vi "Main.vi"() -> ()   [LabVIEW 2019]
uses:
  03 DQMH Modules/SME_Data_Acquisition/SME_Data_Acquisition.lvlib
  03 DQMH Modules/SME_Report/SME_Report.lvlib
panel:
  out "MainTitle":string="SME Client Application"
  in  "Close":bool
  in  "Analysis":bool
  in  "DAQ":bool
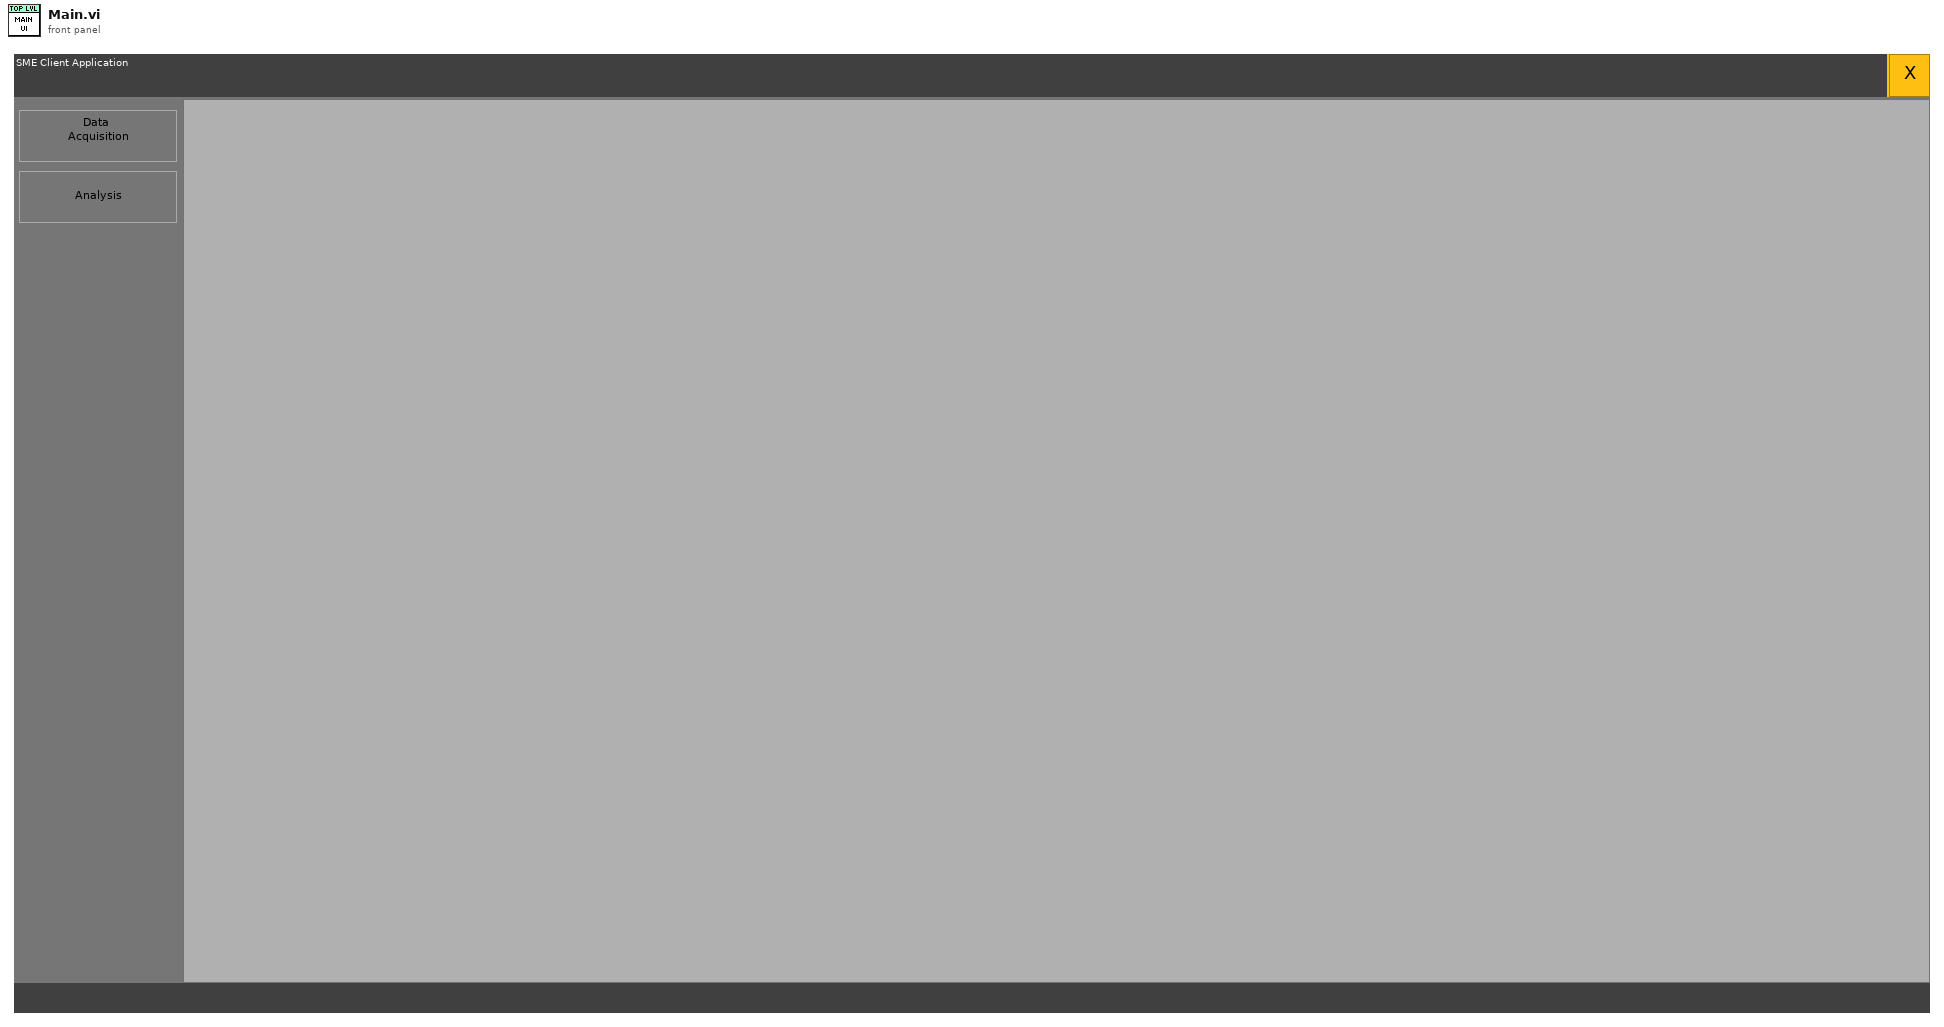
[diagram p1: front panel]
types:
  T1 = enum32{"Invalid", "Standard", "Closed", "Hidden", "Minimized", "Maximized"}
  T2 = enum32{"invalid app kind", "Development System", "Run Time System", "Student Edition", "Embedded LabVIEW", "Evaluation", "Custom"}
  T3 = cluster{"Core":cluster{"Current VI Reference":refnum<vi>, "Close Panel on Exit?":bool}, "MainTitle":refnum<vi>, "SubPanel":refnum<vi>}
  T4 = cluster{"Current VI Reference":refnum<vi>, "Close Panel on Exit?":bool}
  T5 = typedef "LVRectTypeDef.ctl" = cluster{"Left":i16, "Top":i16, "Right":i16, "Bottom":i16}
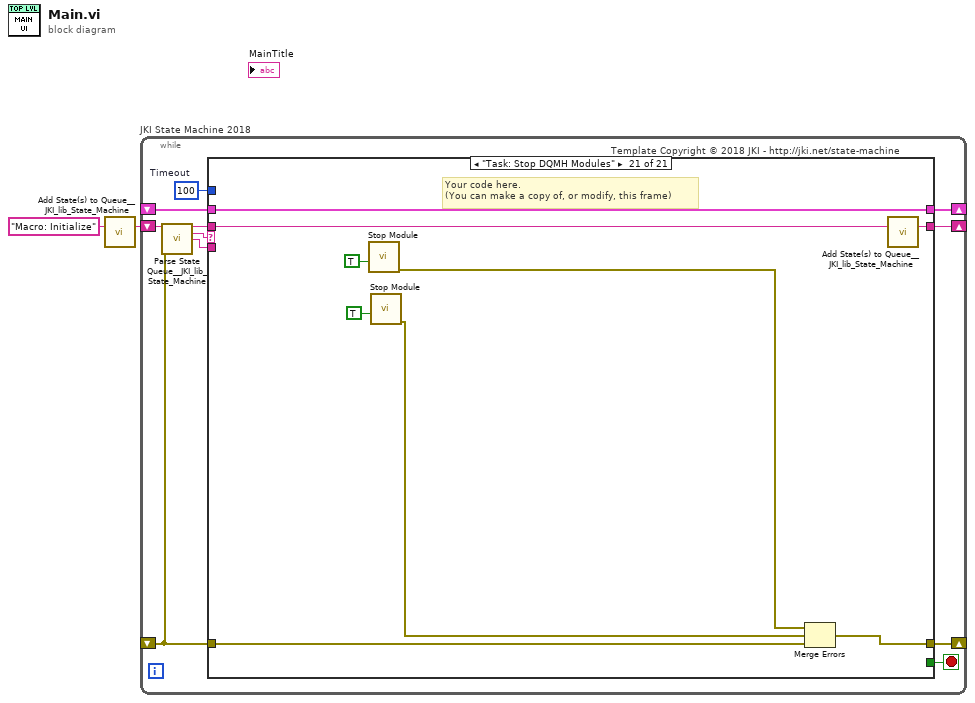
[diagram p0: block diagram]
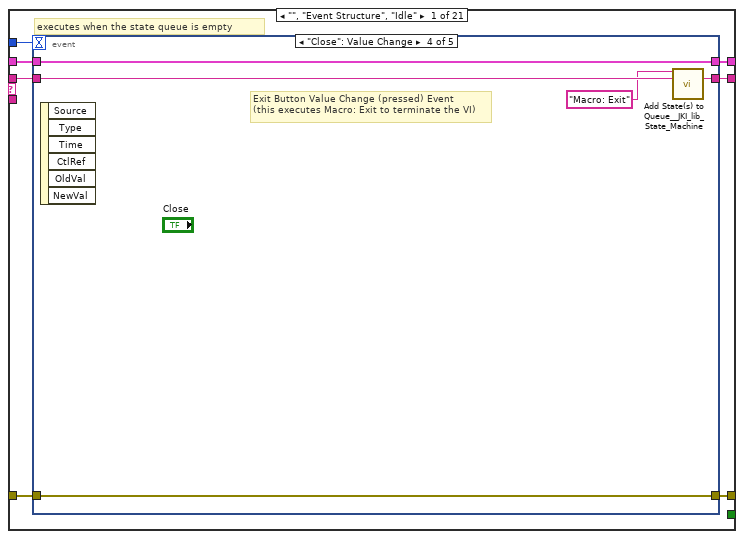
[diagram p2: hidden frame]
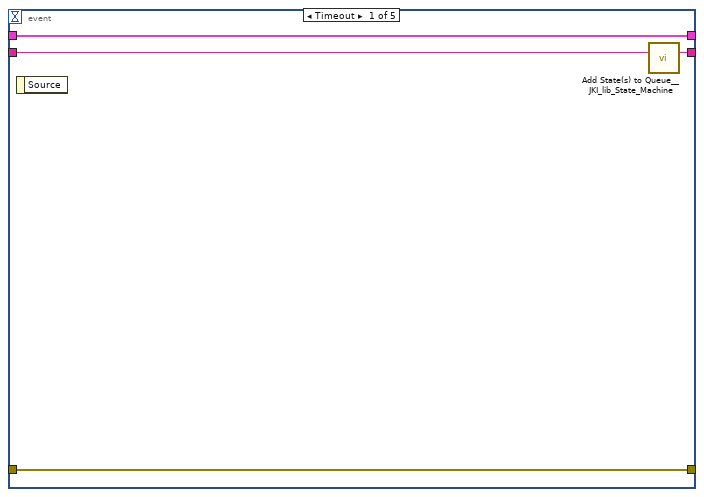
[diagram p3: hidden frame]
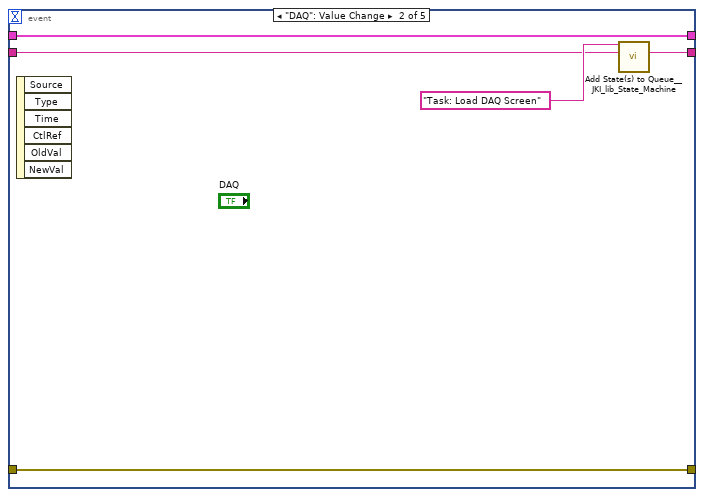
[diagram p4: hidden frame]
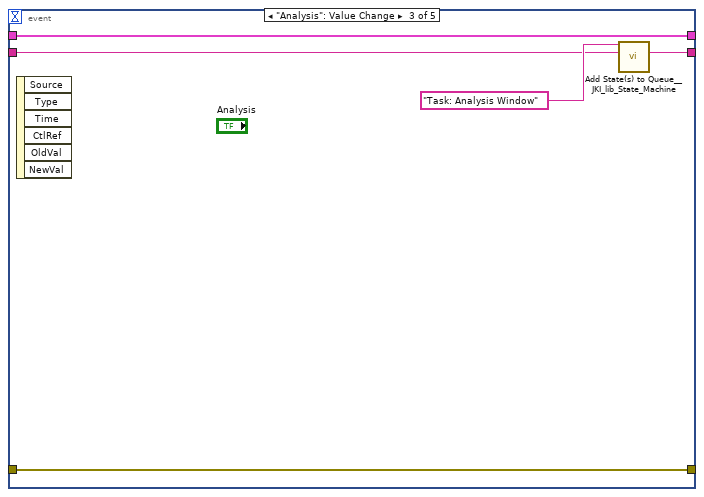
[diagram p5: hidden frame]
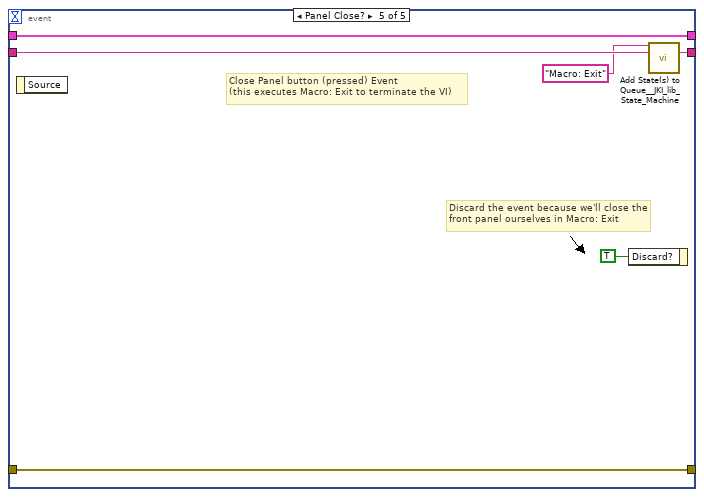
[diagram p6: hidden frame]
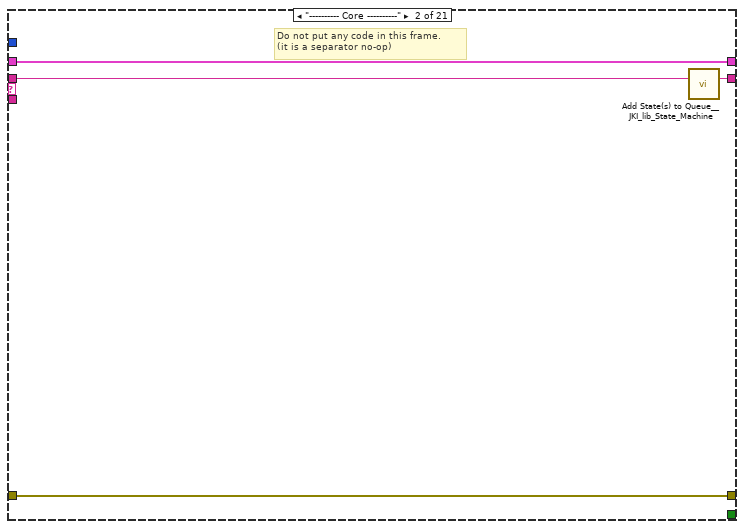
[diagram p7: hidden frame]
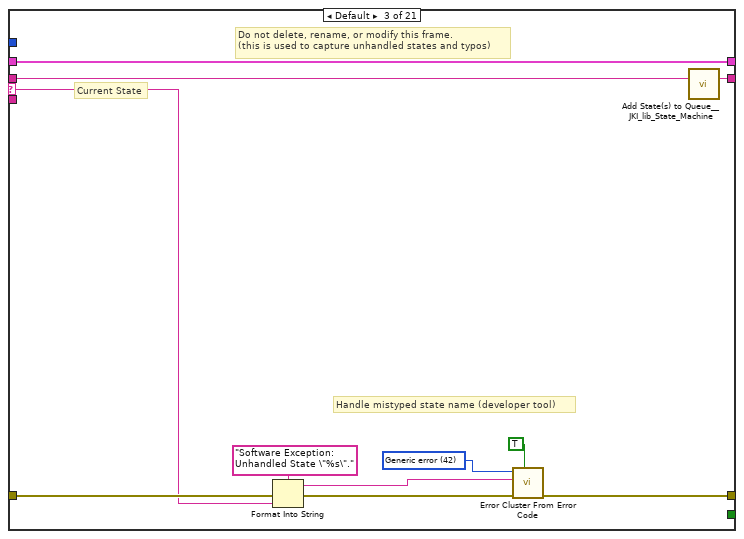
[diagram p8: hidden frame]
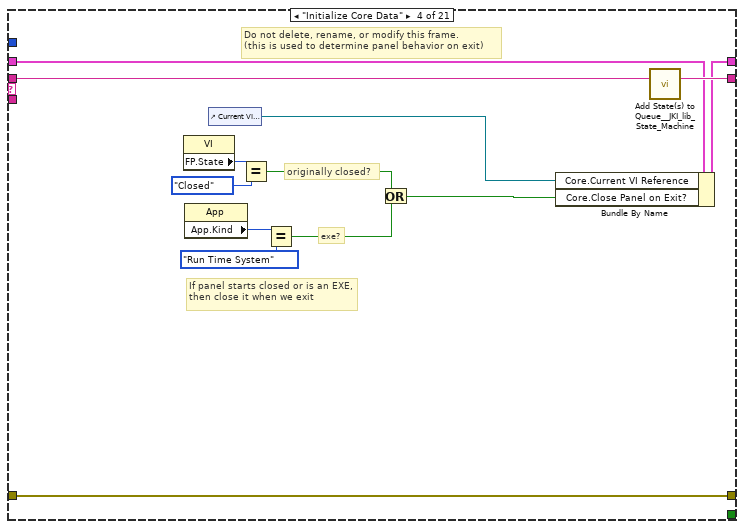
[diagram p9: hidden frame]
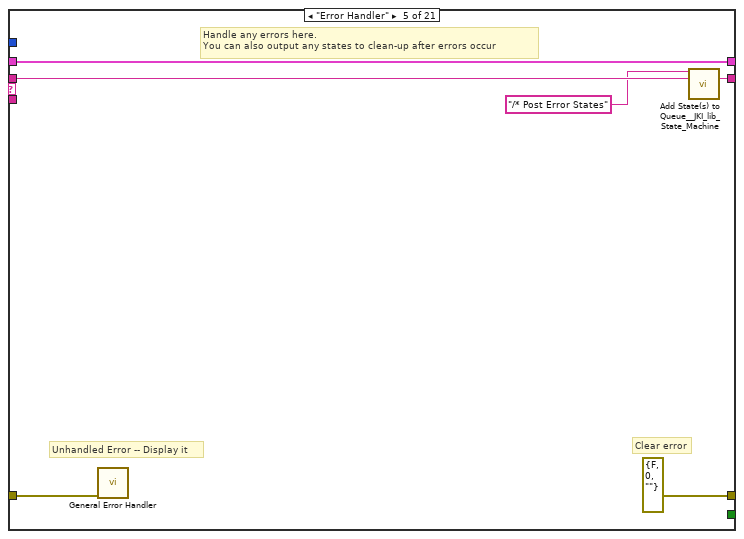
[diagram p10: hidden frame]
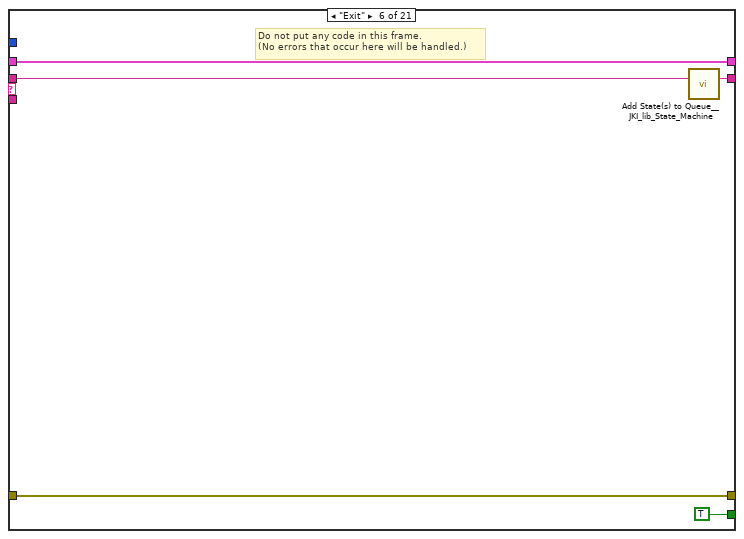
[diagram p11: hidden frame]
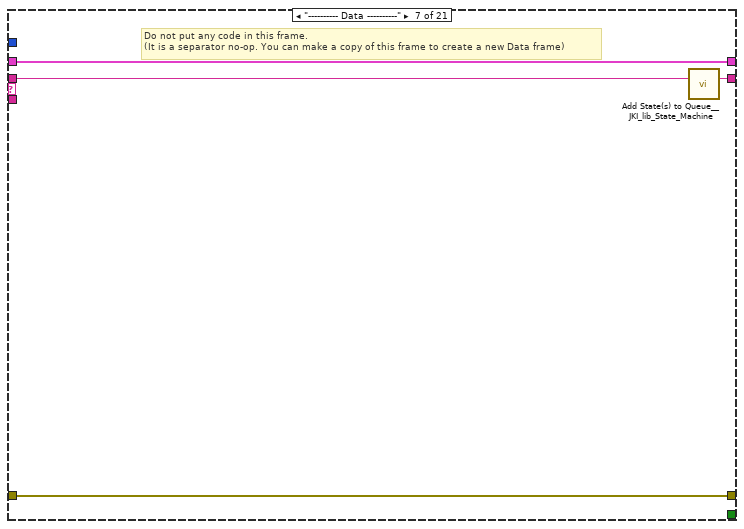
[diagram p12: hidden frame]
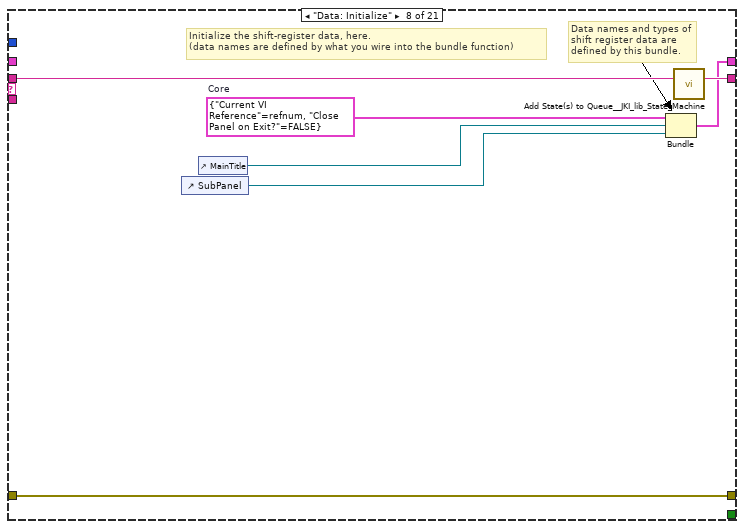
[diagram p13: hidden frame]
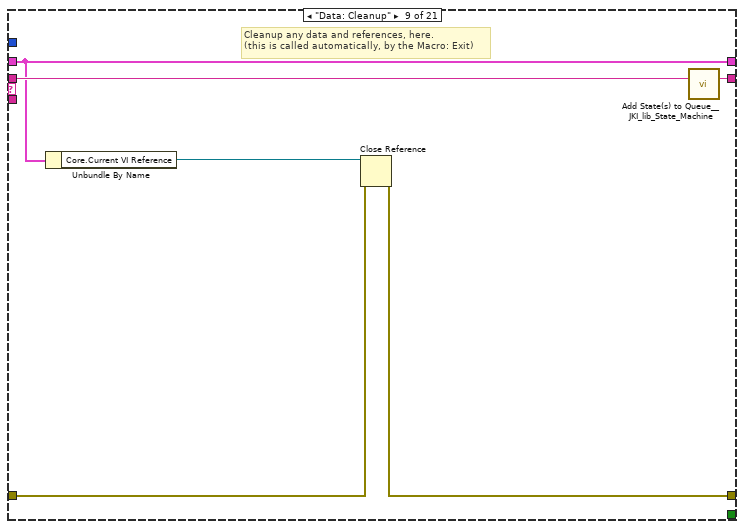
[diagram p14: hidden frame]
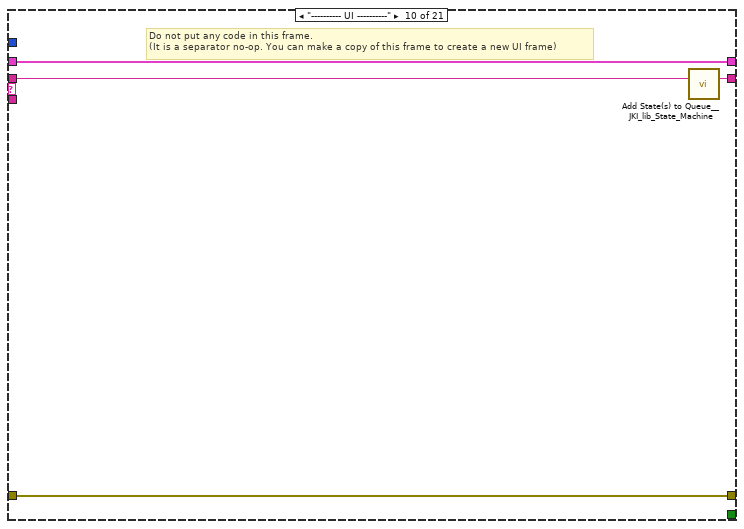
[diagram p15: hidden frame]
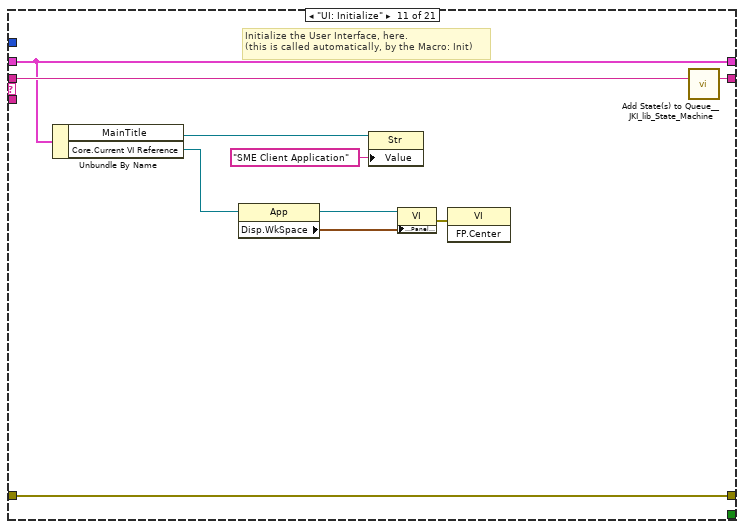
[diagram p16: hidden frame]
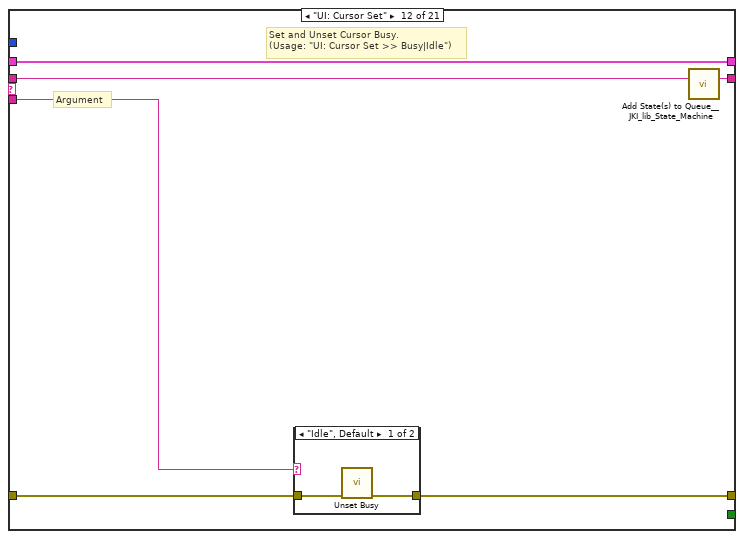
[diagram p17: hidden frame]
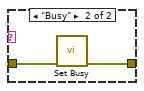
[diagram p18: hidden frame]
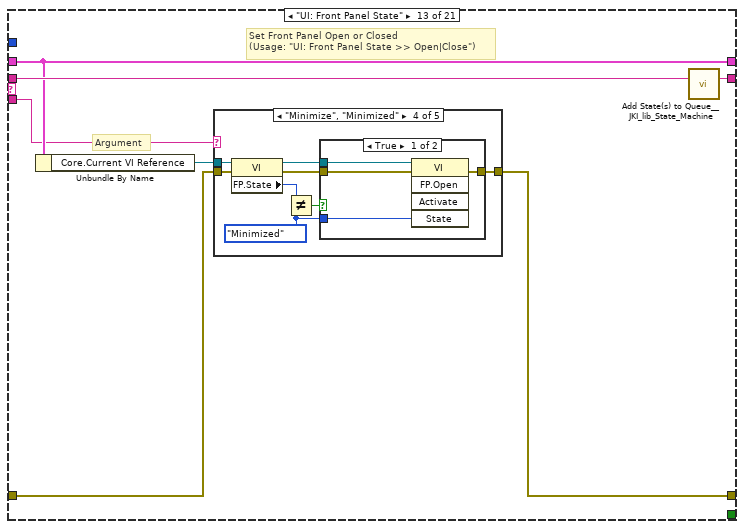
[diagram p19: hidden frame]
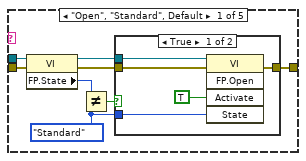
[diagram p20: hidden frame]
diagram:
  n1 = call <vilib>:"Add State(s) to Queue__JKI_lib_State_Machine.vi"("State(s) in (\"\")"="Macro: Initialize") -> ("States Out"=w2:string)  [unwired: 14 in]
  n2 = while "JKI State Machine 2018" {
    shift-right: [w6] -> _
    shift-left: _ -> [w5]
    shift-right: [w9] -> _
    shift-left: _ -> [w3]
    shift-right: [w8] -> _
    shift-left: w2 -> [w10]
    stop <- w7 stop-if-true
    w4 = 100  # Timeout
    # "Template Copyright © 2018 JKI - http://jki.net/state-machine"
    n3 = call <vilib>:"Parse State Queue__JKI_lib_State_Machine.vi"("State Queue"=w10, "Error In (no error)"=w3) -> ("Remaining States"=w12:string, "Current State"=w13:string, "Arguments"=w11:string)  [unwired: 11 in]
    n4 = case shown="\"Task: Stop DQMH Modules\"" w13 {
      selector: w13 -> [_ _ w50 _ _ _ _ _ _ _ _ _ _ _ _ _ _ _ _ _ _]
      tunnel: w12 -> [w20 w49 w54 w73 w79 w84 w88 w95 w101 w105 w114 w120 w131 w200 w205 w215 w219 w230 w240 w250 w259]
      tunnel: w11 -> [_ _ _ _ _ _ _ _ _ _ _ w115 w125 _ _ _ _ _ _ _ _]
      tunnel: w5 -> [w18 w46 w52 w66 w76 w82 w85 _ w96 w102 w111 w118 w127 w197 w203 w212 w216 w227 w231 w248 w256]
      tunnel: [w17 w47 w56 w70 errorcluster {"status"=FALSE, "code"=0, "source"=""} ("error out") w81 w86 w92 w97 w103 w112 w116 w128 w198 w201 w213 w217 w224 w238 w247 w255] -> w9
      tunnel: w3 -> [w16 w47 w55 w70 w75 w81 w86 w92 w98 w103 w112 w117 w129 w198 w201 w213 w217 w228 w238 w246 w257]
      tunnel: [w19 w48 w53 w72 w78 w83 w87 w94 w100 w104 w113 w119 w130 w199 w204 w214 w218 w229 w239 w249 w258] -> w8
      tunnel: [_ _ _ _ _ TRUE _ _ _ _ _ _ _ _ _ _ _ _ _ _ _] -> w7
      tunnel: [w15 w46 w52 w71 w76 w82 w85 w93 w96 w102 w111 w118 w127 w197 w203 w212 w216 w227 w231 w248 w256] -> w6
      tunnel: w4 -> [w14 _ _ _ _ _ _ _ _ _ _ _ _ _ _ _ _ _ _ _ _]
      frame "", "Event Structure", "Idle" {
        # "executes when the state queue is empty"
        n5 = event shown="[3] \"Close\": Value Change" {
          selector: _ -> [_ _ _ _ _]
          dyn-events: _ -> [_ _ _ _ _]
          timeout: w14 -> [_ _ _ _ _]
          tunnel: w20 -> [w24 w26 w31 w39 w45]
          tunnel: [w23 w27 w32 w38 w44] -> w19
          tunnel: w18 -> [w21 w29 w34 w36 w42]
          tunnel: [w22 w25 w30 w37 w43] -> w17
          tunnel: w16 -> [w22 w25 w30 w37 w43]
          tunnel: [w21 w29 w34 w36 w42] -> w15
          event Timeout {
            n6 = event-data() -> ()  [unwired: 1 in, 1 out]
            n7 = call <vilib>:"Add State(s) to Queue__JKI_lib_State_Machine.vi"("State(s) in (\"\")"=w24) -> ("States Out"=w23:string)  [unwired: 14 in]
          }
          event "DAQ": Value Change {
            n8 = event-data() -> ()  [unwired: 1 in, 6 out]
            n9 = call <vilib>:"Add State(s) to Queue__JKI_lib_State_Machine.vi"("State(s) in Front (\"\")"="Task: Load DAQ Screen", "State(s) in (\"\")"=w26) -> ("States Out"=w27:string)  [unwired: 13 in]
          }
          event "Analysis": Value Change {
            n10 = event-data() -> ()  [unwired: 1 in, 6 out]
            n11 = call <vilib>:"Add State(s) to Queue__JKI_lib_State_Machine.vi"("State(s) in Front (\"\")"="Task: Analysis Window", "State(s) in (\"\")"=w31) -> ("States Out"=w32:string)  [unwired: 13 in]
          }
          event "Close": Value Change {
            # "Exit Button Value Change (pressed) Event\n(this executes Macro: Exit to terminate the VI)"
            n12 = event-data() -> ()  [unwired: 1 in, 6 out]
            n13 = call <vilib>:"Add State(s) to Queue__JKI_lib_State_Machine.vi"("State(s) in Front (\"\")"="Macro: Exit", "State(s) in (\"\")"=w39) -> ("States Out"=w38:string)  [unwired: 13 in]
          }
          event Panel Close? {
            # "Discard the event because we'll close the front panel ourselves in Macro: Exit"
            # "Close Panel button (pressed) Event\n(this executes Macro: Exit to terminate the VI)"
            n14 = event-data() -> ()  [unwired: 1 in, 1 out]
            n15 = event-data("Discard?"=TRUE) -> ()  [unwired: 1 in, 1 out]
            n16 = call <vilib>:"Add State(s) to Queue__JKI_lib_State_Machine.vi"("State(s) in Front (\"\")"="Macro: Exit", "State(s) in (\"\")"=w45) -> ("States Out"=w44:string)  [unwired: 13 in]
          }
        }
      }
      frame "---------- Core ----------" {
        # "Do not put any code in this frame.\n(it is a separator no-op)"
        n17 = call <vilib>:"Add State(s) to Queue__JKI_lib_State_Machine.vi"("State(s) in (\"\")"=w49) -> ("States Out"=w48:string)  [unwired: 14 in]
      }
      frame Default {
        w59 = 42 items=["No error", "Argument error", "Memory is full", "Out of zone", "End of file", "File already open", "Generic file I/O error", "File not found", "File permission error", "Disk is full", "Duplicate path", "Too many files open", "System feature not enabled", "Resource file not found", "Cannot add resource", "Resource not found", "Image not found", "Image memory error", "Pen does not exist", "Config type invalid", "Config token not found", "Config parse error", "Config memory error", "Bad external code format", "Bad external code offset", "External code not present", "Null window", "Destroy window error", "Null menu", "Print aborted", "Bad print record", "Print driver error", "Windows error during printing", "Memory error during printing", "Print dialog error", "Generic print error", "Invalid device refnum", "Device not found", "Device parameter error", "Device unit error", "Cannot open device", "Device call aborted", "Generic error", "Cancelled by user", "Object ID too low", "Object ID too high", "Object not in heap", "Unknown heap", "Unknown object (invalid DefProc)", "Unknown object (DefProc not in table)", "Message out of range", "Invalid (null) method", "Unknown message", "Manager call not supported", "Bad address", "Network operation in progress", "Network operation timed out", "Connection is busy", "Network attribute not supported", "Network error", "Address in use", "System out of memory", "Connection aborted", "Connection refused", "Not connected", "Already connected", "Connection closed", "Initialization error (interapplication manager)", "Bad occurrence", "Wait on unbound occurrence handler", "Occurrence queue overflow", "Datalog type conflict", "Unused", "Unrecognized type (interapplication manager)", "Memory corrupt", "Failed to make temporary DLL", "Old CIN version", "Drag socket not found", "Failed to load drop-object", "Failed to register OLE object", "Failed to release OLE object", "Format specifier type mismatch", "Unknown format specifier", "Too few format specifiers", "Too many format specifiers", "Scan failed", "Newer CIN version", "Error converting to variant", "Runtime menu error", "Password tampered", "Variant attribute not found", "Incompatible variant data type", "Event data is not available", "Event Store is not present", "Occurrence is not found", "Event Queue is not created", "Event info is not available", "Refnum passed is NULL", "Error retrieving Class GUID", "Error retrieving CoClass GUID", "Error retrieving TypeLib GUID.", "Bad built application magic bytes.", "Specific driver is different from the specific driver associated with the Logical Name.", "There is no session opened to the class driver.", "Max Error", "MAX - Error with config objects", "MAX - Error loading configuration", "MAX - Group not supported"]
        # "Current State"
        # "Do not delete, rename, or modify this frame.\n(this is used to capture unhandled states and typos)"
        # "Handle mistyped state name (developer tool)"
        n18 = Format Into String(format string="Software Exception: Unhandled State \"%s\"." ("message"), error in=w55, w50) -> (resulting string=w58:string, error out=w57:errorcluster)  [unwired: 1 in]
        n19 = call <vilib>:"Error Cluster From Error Code.vi"("show call chain? (False)"=TRUE, "error in (no error)"=w57, "error message (\"\")"=w58, "error code (0)"=w59) -> ("error out"=w56:errorcluster)  [unwired: 5 in]
        n20 = call <vilib>:"Add State(s) to Queue__JKI_lib_State_Machine.vi"("State(s) in (\"\")"=w54) -> ("States Out"=w53:string)  [unwired: 14 in]
      }
      frame "Initialize Core Data" {
        # "Do not delete, rename, or modify this frame.\n(this is used to determine panel behavior on exit)"
        # "originally closed?"
        # "exe?"
        # "If panel starts closed or is an EXE, then close it when we exit"
        n21 = property class="VI"() -> ("FP.State"=w63:T1)  [unwired: 2 in, 2 out]
        n22 = property class="App"() -> ("App.Kind"=w69:T2)  [unwired: 2 in, 2 out]
        n23 = control-ref of="Current VI Reference"() -> (w64:refnum<vi>)
        n24 = Equal?(x=w63, y=T1."Closed" ("Front Panel Window:State")) -> (x = y?=w61:bool)
        n25 = Equal?(x=w69, y=T2."Run Time System" ("Application:Kind")) -> (x = y?=w67:bool)
        n26 = Or(x=w61, y=w67) -> (x .or. y?=w65:bool)
        n27 = Bundle By Name(cluster=w66, "Core.Current VI Reference"=w64, "Core.Close Panel on Exit?"=w65) -> (w71:T3)
        n28 = call <vilib>:"Add State(s) to Queue__JKI_lib_State_Machine.vi"("State(s) in (\"\")"=w73) -> ("States Out"=w72:string)  [unwired: 14 in]
      }
      frame "Error Handler" {
        # "Unhandled Error -- Display it"
        # "Handle any errors here.\nYou can also output any states to clean-up after errors occur"
        # "Clear error"
        n29 = call <vilib>:"General Error Handler.vi"("error in (no error)"=w75) -> ()  [unwired: 10 in, 5 out]
        n30 = call <vilib>:"Add State(s) to Queue__JKI_lib_State_Machine.vi"("State(s) in Front (\"\")"="/* Post Error States", "State(s) in (\"\")"=w79) -> ("States Out"=w78:string)  [unwired: 13 in]
      }
      frame "Exit" {
        # "Do not put any code in this frame.\n(No errors that occur here will be handled.)"
        n31 = call <vilib>:"Add State(s) to Queue__JKI_lib_State_Machine.vi"("State(s) in (\"\")"=w84) -> ("States Out"=w83:string)  [unwired: 14 in]
      }
      frame "---------- Data ----------" {
        # "Do not put any code in this frame.\n(It is a separator no-op. You can make a copy of this frame to create a new Data frame)"
        n32 = call <vilib>:"Add State(s) to Queue__JKI_lib_State_Machine.vi"("State(s) in (\"\")"=w88) -> ("States Out"=w87:string)  [unwired: 14 in]
      }
      frame "Data: Initialize" {
        w91 = T4 {"Current VI Reference"=refnum, "Close Panel on Exit?"=FALSE}  # Core
        # "Data names and types of shift register data are defined by this bundle."
        # "Initialize the shift-register data, here.\n(data names are defined by what you wire into the bundle function)"
        n33 = control-ref of="SubPanel"() -> (w90:refnum<vi>)
        n34 = control-ref of="MainTitle"() -> (w89:refnum<vi>)
        n35 = Bundle("Core"=w91, "MainTitle"=w89, "SubPanel"=w90) -> (w93:T3)  [unwired: 1 in]
        n36 = call <vilib>:"Add State(s) to Queue__JKI_lib_State_Machine.vi"("State(s) in (\"\")"=w95) -> ("States Out"=w94:string)  [unwired: 14 in]
      }
      frame "Data: Cleanup" {
        # "Cleanup any data and references, here.\n(this is called automatically, by the Macro: Exit)"
        n37 = Unbundle By Name(w96) -> ("Core.Current VI Reference"=w99:refnum<vi>)
        n38 = Close Reference(reference=w99, error in (no error)=w98) -> (error out=w97:errorcluster)
        n39 = call <vilib>:"Add State(s) to Queue__JKI_lib_State_Machine.vi"("State(s) in (\"\")"=w101) -> ("States Out"=w100:string)  [unwired: 14 in]
      }
      frame "---------- UI ----------" {
        # "Do not put any code in this frame.\n(It is a separator no-op. You can make a copy of this frame to create a new UI frame)"
        n40 = call <vilib>:"Add State(s) to Queue__JKI_lib_State_Machine.vi"("State(s) in (\"\")"=w105) -> ("States Out"=w104:string)  [unwired: 14 in]
      }
      frame "UI: Initialize" {
        # "Initialize the User Interface, here.\n(this is called automatically, by the Macro: Init)"
        n41 = Unbundle By Name(w111) -> ("MainTitle"=w110:refnum<vi>, "Core.Current VI Reference"=w106:refnum<vi>)
        n42 = property on="Property Node" class="App"() -> ("Disp.WkSpace"=w107:T5)  [unwired: 2 in, 2 out]
        n43 = property class="Str"(reference=w110, "Value"="SME Client Application") -> ()  [unwired: 1 in, 2 out]
        n44 = property on="Property Node" class="VI"(reference=w106, "Front Panel.PanelBounds"=w107) -> (error out=w108:errorcluster)  [unwired: 1 in, 1 out]
        n45 = invoke class="VI" method="FP.Center"(error in=w108) -> ()  [unwired: 2 in, 3 out]
        n46 = call <vilib>:"Add State(s) to Queue__JKI_lib_State_Machine.vi"("State(s) in (\"\")"=w114) -> ("States Out"=w113:string)  [unwired: 14 in]
      }
      frame "UI: Cursor Set" {
        # "Argument"
        # "Set and Unset Cursor Busy.\n(Usage: \"UI: Cursor Set >> Busy|Idle\")"
        n47 = case shown="\"Idle\", Default" w115 {
          tunnel: w117 -> [w122 w124]
          tunnel: [w121 w123] -> w116
          frame "Idle", Default {
            n48 = call <vilib>:"Unset Busy.vi"("error in (no error)"=w122) -> ("error out"=w121:errorcluster)  [unwired: 10 in]
          }
          frame "Busy" {
            n49 = call <vilib>:"Set Busy.vi"("error in (no error)"=w124) -> ("error out"=w123:errorcluster)  [unwired: 9 in, 1 out]
          }
        }
        n50 = call <vilib>:"Add State(s) to Queue__JKI_lib_State_Machine.vi"("State(s) in (\"\")"=w120) -> ("States Out"=w119:string)  [unwired: 14 in]
      }
      frame "UI: Front Panel State" {
        # "Argument"
        # "Set Front Panel Open or Closed\n(Usage: \"UI: Front Panel State >> Open|Close\")"
        n51 = Unbundle By Name(w127) -> ("Core.Current VI Reference"=w126:refnum<vi>)
        n52 = case shown="\"Minimize\", \"Minimized\"" w125 {
          tunnel: w129 -> [w137 w152 w163 w176 w189]
          tunnel: [w139 w153 w165 w178 w191] -> w128
          tunnel: w126 -> [w138 w150 w164 w177 w190]
          frame "Open", "Standard", Default {
            w132 = T1."Standard" ("State")
            n53 = property class="VI"(reference=w138, error in=w137) -> (reference out=w135:refnum<vi>, error out=w136:errorcluster, "FP.State"=w134:T1)
            n54 = Not Equal?(x=w134, y=w132) -> (x != y?=w133:bool)
            n55 = case shown="True" w133 {
              tunnel: [w143 w145] -> w139
              tunnel: w136 -> [w142 w145]
              tunnel: w135 -> [w141 _]
              tunnel: w132 -> [w140 _]
              frame True {
                n56 = invoke class="VI" method="FP.Open"(reference=w141, error in=w142, "Activate"=TRUE, "State"=w140) -> (error out=w143:errorcluster)  [unwired: 1 in, 4 out]
              }
              frame False {
              }
            }
          }
          frame "Close", "Closed" {
            n57 = property class="VI"(reference=w150, error in=w152) -> (reference out=w149:refnum<vi>, error out=w151:errorcluster, "FP.State"=w147:T1)
            n58 = Not Equal?(x=w147, y=T1."Closed" ("Front Panel Window:State")) -> (x != y?=w146:bool)
            n59 = case shown="True" w146 {
              tunnel: [w154 w157] -> w153
              tunnel: w151 -> [w154 w156]
              tunnel: w149 -> [_ w155]
              frame False {
              }
              frame True {
                n60 = invoke class="VI" method="FP.Close"(reference=w155, error in=w156) -> (error out=w157:errorcluster)  [unwired: 1 in, 2 out]
              }
            }
          }
          frame "Hidden", "Hide" {
            w158 = T1."Hidden" ("State")
            n61 = property class="VI"(reference=w164, error in=w163) -> (reference out=w161:refnum<vi>, error out=w162:errorcluster, "FP.State"=w160:T1)
            n62 = Not Equal?(x=w160, y=w158) -> (x != y?=w159:bool)
            n63 = case shown="True" w159 {
              tunnel: [w169 w170] -> w165
              tunnel: w162 -> [w168 w170]
              tunnel: w161 -> [w167 _]
              tunnel: w158 -> [w166 _]
              frame True {
                n64 = invoke class="VI" method="FP.Open"(reference=w167, error in=w168, "State"=w166) -> (error out=w169:errorcluster)  [unwired: 2 in, 4 out]
              }
              frame False {
              }
            }
          }
          frame "Minimize", "Minimized" {
            w171 = T1."Minimized" ("State")
            n65 = property class="VI"(reference=w177, error in=w176) -> (reference out=w174:refnum<vi>, error out=w175:errorcluster, "FP.State"=w173:T1)
            n66 = Not Equal?(x=w173, y=w171) -> (x != y?=w172:bool)
            n67 = case shown="True" w172 {
              tunnel: [w182 w183] -> w178
              tunnel: w175 -> [w181 w183]
              tunnel: w174 -> [w180 _]
              tunnel: w171 -> [w179 _]
              frame True {
                n68 = invoke class="VI" method="FP.Open"(reference=w180, error in=w181, "State"=w179) -> (error out=w182:errorcluster)  [unwired: 2 in, 4 out]
              }
              frame False {
              }
            }
          }
          frame "Maximize", "Maximized" {
            w184 = T1."Maximized" ("State")
            n69 = property class="VI"(reference=w190, error in=w189) -> (reference out=w187:refnum<vi>, error out=w188:errorcluster, "FP.State"=w186:T1)
            n70 = Not Equal?(x=w186, y=w184) -> (x != y?=w185:bool)
            n71 = case shown="True" w185 {
              tunnel: [w195 w196] -> w191
              tunnel: w188 -> [w194 w196]
              tunnel: w187 -> [w193 _]
              tunnel: w184 -> [w192 _]
              frame True {
                n72 = invoke class="VI" method="FP.Open"(reference=w193, error in=w194, "State"=w192) -> (error out=w195:errorcluster)  [unwired: 2 in, 4 out]
              }
              frame False {
              }
            }
          }
        }
        n73 = call <vilib>:"Add State(s) to Queue__JKI_lib_State_Machine.vi"("State(s) in (\"\")"=w131) -> ("States Out"=w130:string)  [unwired: 14 in]
      }
      frame "---------- Macro ----------" {
        # "Do not put any code in this frame.\n(It is a separator no-op. You can make a copy of this frame to create a new Macro frame)"
        n74 = call <vilib>:"Add State(s) to Queue__JKI_lib_State_Machine.vi"("State(s) in (\"\")"=w200) -> ("States Out"=w199:string)  [unwired: 14 in]
      }
      frame "Macro: Initialize" {
        # "Initialization Macro\n(This is called once, when the VI starts)"
        n75 = call <vilib>:"Add State(s) to Queue__JKI_lib_State_Machine.vi"("State(s) in Front (\"\")"="Data: Initialize\nInitialize Core Data\nUI: Initialize\nUI: Front Panel State >> Open\nTask: Start DQMH Modules", "State(s) in (\"\")"=w205) -> ("States Out"=w204:string)  [unwired: 13 in]
      }
      frame "Macro: Exit" {
        # "Exit Macro\n(This is called once, when the VI exits)"
        n76 = Unbundle By Name(w212) -> ("Core.Close Panel on Exit?"=w211:bool)
        n77 = Select(t="Task: Stop DQMH Modules\nUI: Front Panel State >> Close", s=w211, f="") -> (s? t:f=w208:string)
        n78 = call <vilib>:"Add State(s) to Queue__JKI_lib_State_Machine.vi"("State(s) in (\"\")"=w208, "State(s) at Back (\"\")"="Task: Stop DQMH Modules\nData: Cleanup\nExit") -> ("States Out"=w206:string)  [unwired: 13 in]
        n79 = call <vilib>:"Add State(s) to Queue__JKI_lib_State_Machine.vi"("State(s) in Front (\"\")"=w206, "State(s) in (\"\")"=w215) -> ("States Out"=w214:string)  [unwired: 13 in]
      }
      frame "---------- Task ----------" {
        # "Template Separator\n(You can make a copy of, or modify, this frame)"
        n80 = call <vilib>:"Add State(s) to Queue__JKI_lib_State_Machine.vi"("State(s) in (\"\")"=w219) -> ("States Out"=w218:string)  [unwired: 14 in]
      }
      frame "Task: Start DQMH Modules" {
        # "Your code here.\n(You can make a copy of, or modify, this frame)"
        n81 = call "Start Module.vi"() -> ("error out"=w226:errorcluster, "Wait for Event Sync?"=w225:bool)  [unwired: 8 in, 2 out]
        n82 = call "Start Module.vi"() -> ("error out"=w222:errorcluster, "Wait for Event Sync?"=w221:bool)  [unwired: 8 in, 2 out]
        n83 = call "Synchronize Module Events.vi"("error in"=w226, "Wait for Event Sync?"=w225) -> ("error out"=w223:errorcluster)  [unwired: 9 in]
        n84 = call "Synchronize Module Events.vi"("error in"=w222, "Wait for Event Sync?"=w221) -> ("error out"=w220:errorcluster)  [unwired: 9 in]
        n85 = Merge Errors(w223, w220, w228) -> (w224:errorcluster)
        n86 = call <vilib>:"Add State(s) to Queue__JKI_lib_State_Machine.vi"("State(s) in (\"\")"=w230) -> ("States Out"=w229:string)  [unwired: 14 in]
      }
      frame "Task: Load DAQ Screen" {
        # "Your code here.\n(You can make a copy of, or modify, this frame)"
        n87 = Unbundle By Name(w231) -> ("SubPanel"=w237:refnum<vi>)
        n88 = property class="SubPnl"(reference=w237) -> (reference out=w235:refnum<vi>, error out=w236:errorcluster, "InsertedVI"=w234:refnum<vi>)  [unwired: 1 in]
        n89 = vi-ref "SME_Data_Acquisition.lvlib:Main.vi"() -> (w232:refnum<vi>)
        n90 = Equal?(x=w232, y=w234) -> (x = y?=w233:bool)
        n91 = case shown="False" w233 {
          tunnel: [w241 w245] -> _
          tunnel: w236 -> [w244 w245]
          tunnel: w235 -> [w242 _]
          tunnel: w232 -> [w243 _]
          frame False {
            n92 = call "Insert SubPanel.vi"("error in (no error)"=w244, "VI Ref"=w243, "Subpanel Ref"=w242) -> ("error out"=w241:errorcluster)  [unwired: 8 in]
          }
          frame True {
          }
        }
        n93 = call <vilib>:"Add State(s) to Queue__JKI_lib_State_Machine.vi"("State(s) in (\"\")"=w240) -> ("States Out"=w239:string)  [unwired: 14 in]
      }
      frame "Task: Analysis Window" {
        # "Template Separator\n(You can make a copy of, or modify, this frame)"
        n94 = call "Show Panel.vi"("error in"=w246) -> ("error out"=w247:errorcluster)  [unwired: 10 in]
        n95 = call <vilib>:"Add State(s) to Queue__JKI_lib_State_Machine.vi"("State(s) in (\"\")"=w250) -> ("States Out"=w249:string)  [unwired: 14 in]
      }
      frame "Task: Stop DQMH Modules" {
        # "Your code here.\n(You can make a copy of, or modify, this frame)"
        n96 = call "Stop Module.vi"("Wait for Module to Stop? (F)"=TRUE) -> ("error out"=w254:errorcluster)  [unwired: 10 in]
        n97 = call "Stop Module.vi"("Wait for Module to Stop? (F)"=TRUE) -> ("error out"=w253:errorcluster)  [unwired: 10 in]
        n98 = Merge Errors(w254, w253, w257) -> (w255:errorcluster)
        n99 = call <vilib>:"Add State(s) to Queue__JKI_lib_State_Machine.vi"("State(s) in (\"\")"=w259) -> ("States Out"=w258:string)  [unwired: 14 in]
      }
    }
  }
